vi "resampled-to-waveform.vi"(10 "resampled data":T1[](array[typedef]) {"resampled signal" format="%.2f"; "times [s]" format="%.2f"}, 11 "current-timestamp":timestamp) -> (3 "waveform data":waveform(dbl)[](array[waveform]))   [LabVIEW 2024]
uses:
  <vilib>/addons/Electrical Power/Power Measurement/subVIs/ep_Resampled Data.ctl
  <vilib>/addons/Electrical Power/Power Measurement/NI_EP_Power Measurement.lvlib
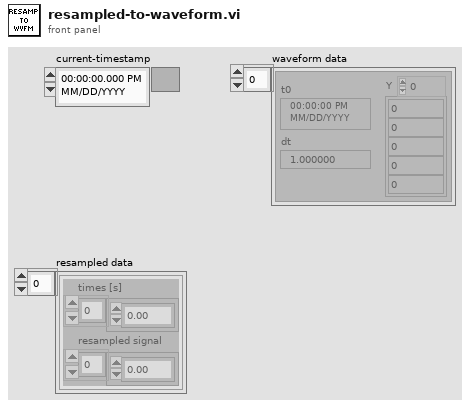
[diagram p1: front panel]
types:
  T1 = typedef "NI_EP_Power Measurement.lvlib/ep_Resampled Data.ctl" = cluster{"times [s]":dbl[], "resampled signal":dbl[]}
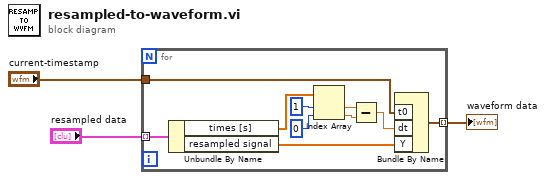
[diagram p0: block diagram]
diagram:
  n1 = for {
    tunnel: "resampled data" -> [w13] mode=indexing
    tunnel: [w6] -> w3 mode=indexing
    tunnel: "current-timestamp" -> [w4]
    n2 = Unbundle By Name(w13) -> ("times [s]"=w5:dbl[], "resampled signal"=w8:dbl[])
    n3 = Index Array(array=w5, index #1=1 ("index"), index #2=0 ("index")) -> (element #1=w11:dbl, element #2=w12:dbl)
    n4 = Subtract(x=w11, y=w12) -> (x-y=w7:dbl)
    n5 = Bundle By Name("t0"=w4, "dt"=w7, "Y"=w8) -> (w6:waveform(dbl))  [unwired: 1 in]
  }
  "waveform data" <- w3
